vi "Timing-Precise Time.vi"(11 "error in (no error)":errorcluster) -> (8 "preciseTime":i64, 15 "error out":errorcluster)   [LabVIEW 2020]
uses:
  kernel32.dll
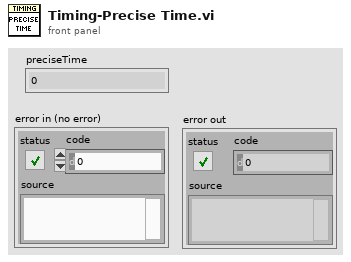
[diagram p1: front panel]
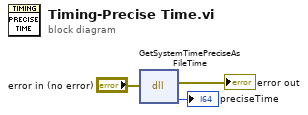
[diagram p0: block diagram]
diagram:
  n1 = dll-call lib="kernel32.dll" fn="GetSystemTimePreciseAsFileTime"(error in="error in (no error)") -> (error out=→"error out":errorcluster, "preciseTime"=→"preciseTime":i64)  [unwired: 4 in, 1 out]
